vi "FOFB Data Archiver Main.vi"() -> ()   [LabVIEW 2011]
uses:
  Types Definitions/Type BPM and PS select cluster.ctl
  <vilib>/Platform/TimedLoop/XDataNode/timing_clust.ctl
  <vilib>/Platform/TimedLoop/XDataNode/nitl_modes.ctl
  <vilib>/Platform/TimedLoop/XDataNode/wakeup.ctl
  <vilib>/Platform/TimedLoop/XDataNode/XDataNode.xnode
  Type Definitions.lvlib
  Controller VIs.lvlib
  <vilib>/Platform/TimedLoop/XDataNode/XDNodeRunTimeDep.lvlib
  File VIs.lvlib
  kernel32.dll
panel:
  out "Slide":dbl(slide)
  out "Next filename":string caption="Registro de dados em:"
  out "Status":bool caption="Registrando dados..."
  in  "Path":path=path "E:/" caption="Diretório de armazenamento"
  in  "Maximum number of files":i32=18900 caption="Máximo número de arquivos:"
  in  "Number of packets per file":i32=1000 caption="Número de pacotes de dados por arquivo:"
  in  "FOFB Controller IP":string="10.0.5.31" caption="IP do controlador do FOFB (PXI):"
  in  "stop":bool
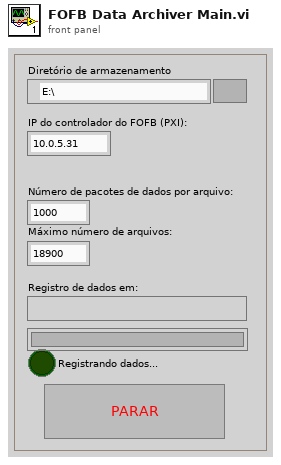
[diagram p1: front panel]
types:
  T1 = typedef "Type Definitions.lvlib/Type BPM and PS select cluster.ctl" = cluster{"BPM index array":u32[], "PS index array ":u32[]}
  T2 = enum16{"Idle", "Wait Connection", "Read Data", "Close Connection"}
  T3 = typedef "XDNodeRunTimeDep.lvlib/timing_clust.ctl" = cluster{"Expected End [f-1]":u64, "Actual End [f-1]":u64, "Finished Late? [f-1]":bool, "Expected End [i-1]":u64, "Actual End [i-1]":u64, "Finished Late? [i-1]":bool, "Expected Start [i]":u64, "Actual Start [i]":u64, "Expected Start [f]":u64, "Actual Start [f]":u64, "Source Name":string, "Structure Name":string, "Period":i64, "Deadline":i64, "Offset":i64, "Start":i64, "Priority":i32, "Timeout":i32, "Mode":T4, "Wakeup Reason":T5, "Error":errorcluster, "Source Type":string, "Secondary Source Type":string, "Global End Time":u64, "Global Start Time":u64, "Frame Duration":u64, "Iteration Duration":u64, "Assigned CPU":i32, "I/O Scan Engine Mode":u32}
  T4 = typedef "XDNodeRunTimeDep.lvlib/nitl_modes.ctl" = enum32{"No Change", "Process missed periods, maintain original phase", "Discard missed periods, maintain original phase", "Process missed periods, ignore original phase", "Discard missed periods, ignore original phase"}
  T5 = typedef "XDNodeRunTimeDep.lvlib/wakeup.ctl" = enum32{"Normal", "Aborted", "Asynchronous wakeup", "Timing source error", "Timed loop error", "Timeout"}
  T6 = enum16{"open", "replace", "create", "open or create", "replace or create", "replace or create with confirmation"}
  T7 = typedef "Type Definitions.lvlib/Type FOFB Parameters.ctl" = cluster{"Network":T8, "Fast Acquisition":T9, "Response Matrix Measurement":T10, "Correction Algorithm":T11, "Acquisition Network":T12, "Actuation Network":T13}
  T8 = typedef "Type Definitions.lvlib/Type Network Configuration.ctl" = cluster{"FOFB Controller IP":string, "LNLS Control Network IP":string, "LNLS Control Network Power Supplies TCP Port":u16, "LNLS Control Network FOFB Configuration TCP Port":u16, "LNLS Control Network BPMs TCP Port":u16, "Data Server TCP Port":u16, "Monitoring Data TCP Port":u16, "Configuration GUI TCP Port":u16, "Storage Data TCP Port":u16, "Fast Command TCP Port":u16, "TCP Listening Timeout":i32, "Request Setpoints Rate":u16}
  T9 = typedef "Type Definitions.lvlib/Type FA Configuration.ctl" = cluster{"Acquisition Period":u32, "Data Buffer Size":u32, "Monitoring Period":u32}
  T10 = typedef "Type Definitions.lvlib/Type Response Matrix Measurement Configuration.ctl" = cluster{"Step Amplitude":dbl, "Time Between Steps":u32, "Step Duration":u32, "Number of Averages":u32}
  T11 = typedef "Type Definitions.lvlib/Type Correction Algorithm Configuration.ctl" = cluster{"Correction Period":u32, "Reference Orbit Path":path, "Response Matrix Path":path, "Correction Matrix Path":path, "PID Horizontal Gain":dbl, "PID Vertical Gain":dbl, "PID Horizontal Integral Time":dbl, "PID Vertical Integral Time":dbl, "PID Horizontal Derivative Time":dbl, "PID Vertical Derivative Time":dbl, "Beam Current FOFB Threshold":dbl, "Decouple H-V":bool, "Use Additional BPM LPF":bool, "BPM LPF Cutoff":dbl}
  T12 = typedef "Type Definitions.lvlib/Type Acquisition Network Configuration.ctl" = cluster{"Chassis Name":string, "Variables":cluster{"Variable Name":string, "Matrix Order":u32, "Location":dbl, "Plane":enum8{"H", "V"}, "On Correction":bool}[]}[]
  T13 = typedef "Type Definitions.lvlib/Type Actuation Network Configuration.ctl" = cluster{"Chassis Name":string, "Variables":cluster{"Variable Name":string, "Matrix Order":u32, "RMM Step Factor":dbl, "Plane":enum8{"H", "V"}, "On Correction":bool, "Kc":dbl, "Ti":dbl, "Td":dbl}[]}[]
  T14 = typedef "Type Definitions.lvlib/Type FOFB Configuration.ctl" = cluster{"FOFB Parameters":T7, "Number of Acquisition Chassis":i32, "Number of Actuation Chassis":i32, "Number of BPM Readings":i32, "BPM Reading Names":string[], "Selected BPM Readings":u32[], "Number of Correctors":i32, "Corrector Names":string[], "Selected Correctors":u32[], "Reference Orbit":dbl[], "Response Matrix":dbl[][], "Correction Matrix":dbl[][], "Acquisition Chassis Names":string[], "Actuation Chassis Names":string[], "Acquisition Variables":cluster{"Variable Name":string, "Chassis Name":string}[], "Actuation Variables":cluster{"Variable Name":string, "Chassis Name":string}[], "PS Matrix Mapping":cluster{u32[]}[], "Inverse PS Matrix Mapping":u32[][], "BPM Matrix Mapping":cluster{u32[]}[], "Inverse BPM Matrix Mapping":u32[][], "Response Matrix Beam Energy (MeV)":dbl, "PID Parameters":T15[], "BPM Planes":enum8{"H", "V"}[], "Corrector Planes":enum8{"H", "V"}[], "RMM Step Factor":dbl[]}
  T15 = typedef "Type Definitions.lvlib/Type PID Parameters.ctl" = cluster{"Kc":fxp<+/-,16,8>, "Ti":fxp<+/-,16,8>, "Td":fxp<+/-,16,8>}
  T16 = enum16{"Standard", "Buffered", "CRLF", "Immediate"}
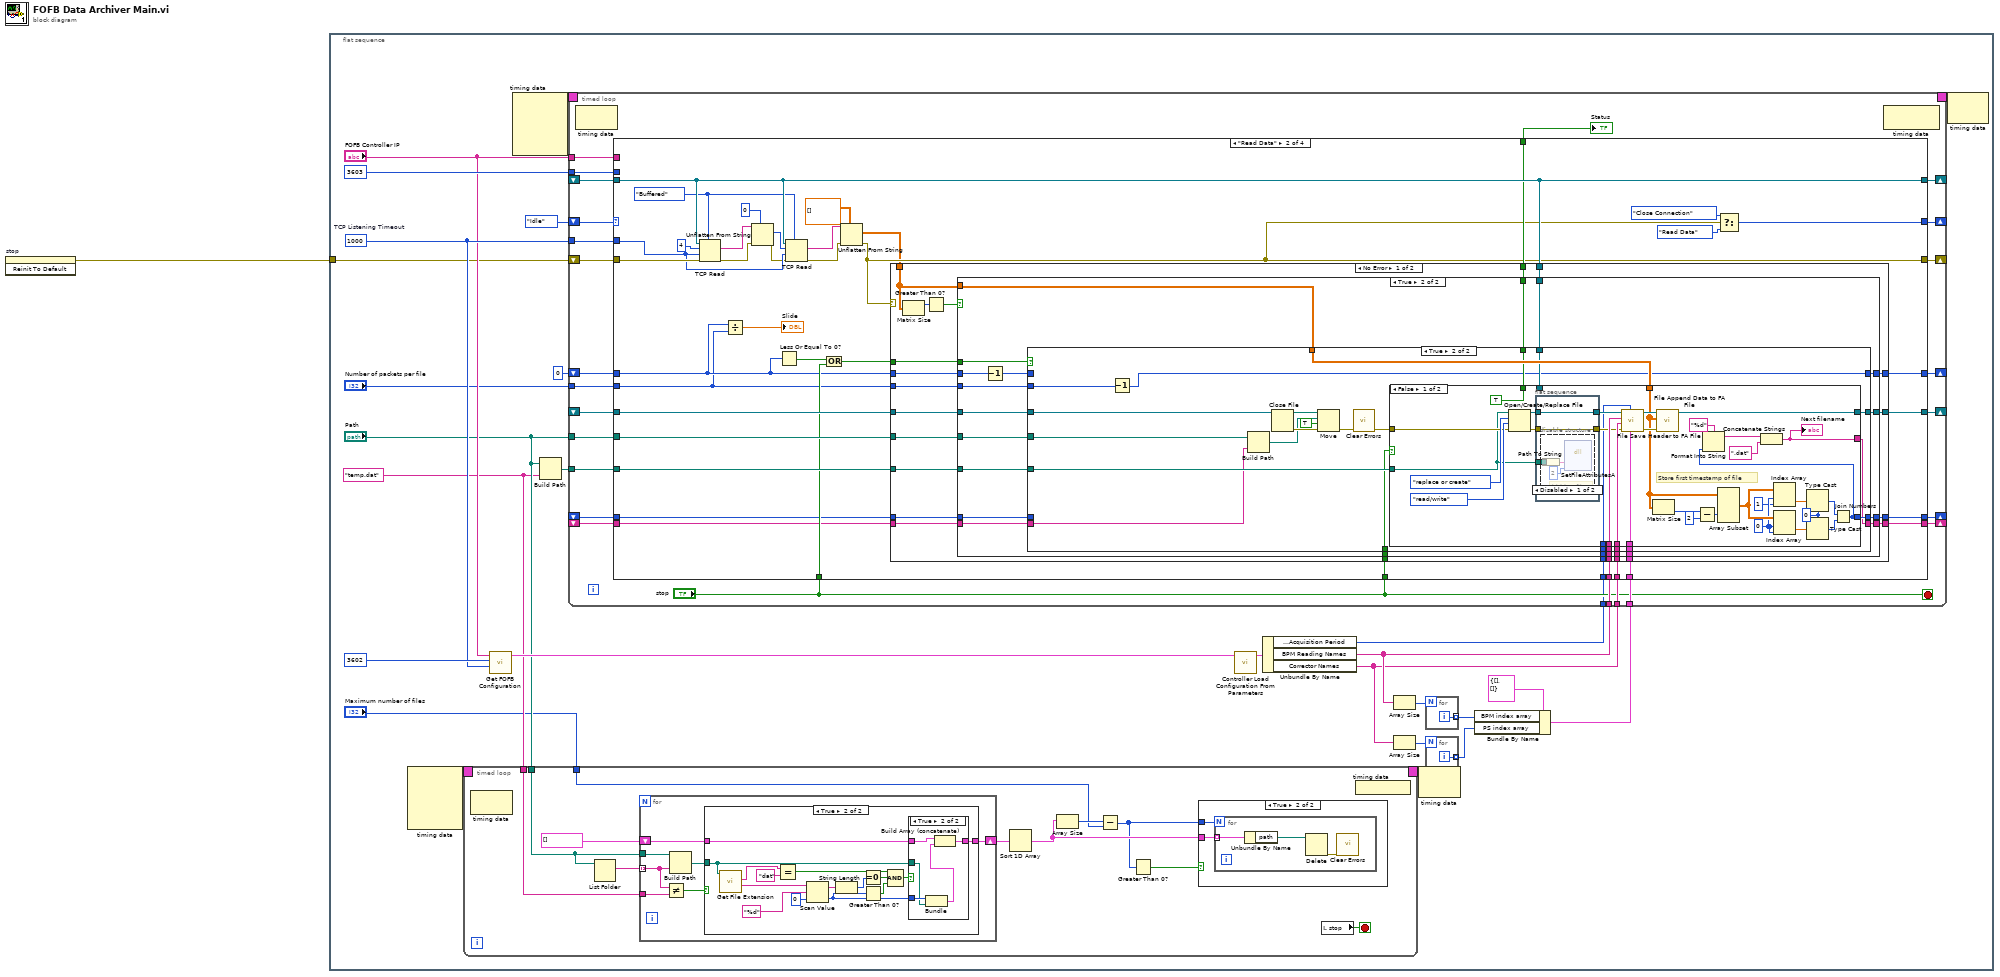
[diagram p0: block diagram]
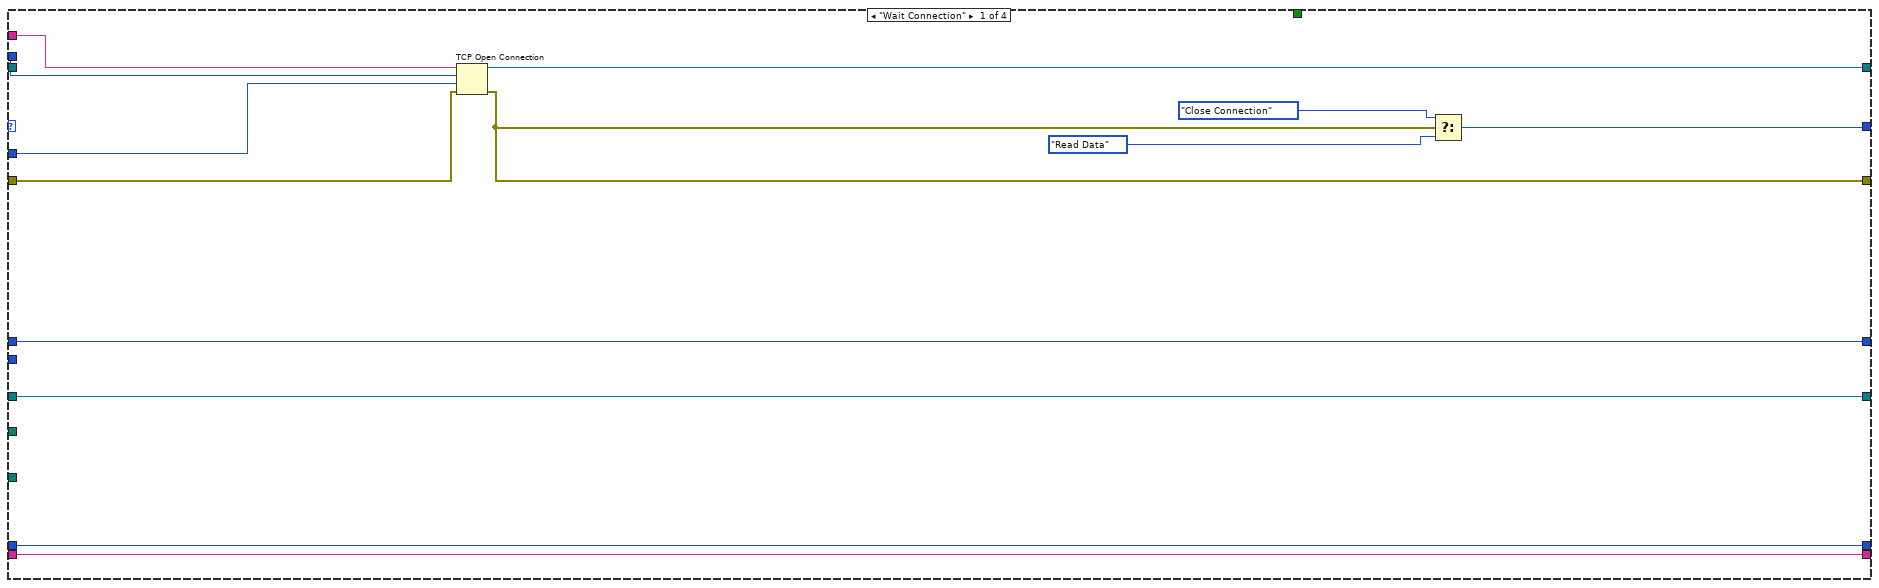
[diagram p2: hidden frame]
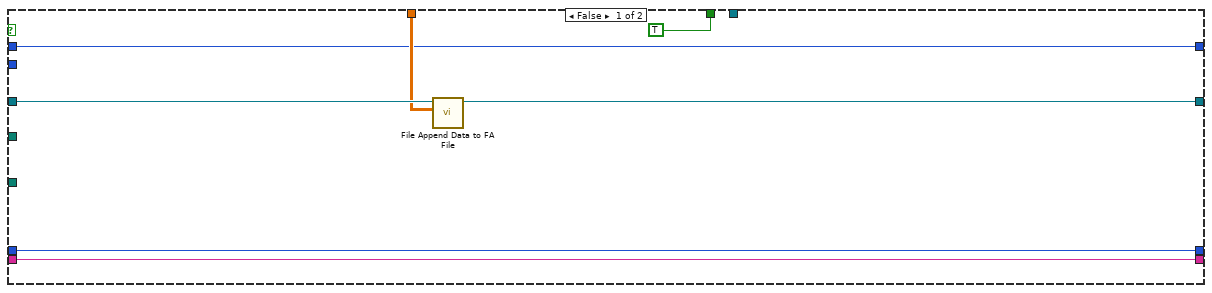
[diagram p4: hidden frame]
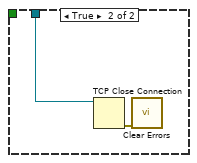
[diagram p6: hidden frame]
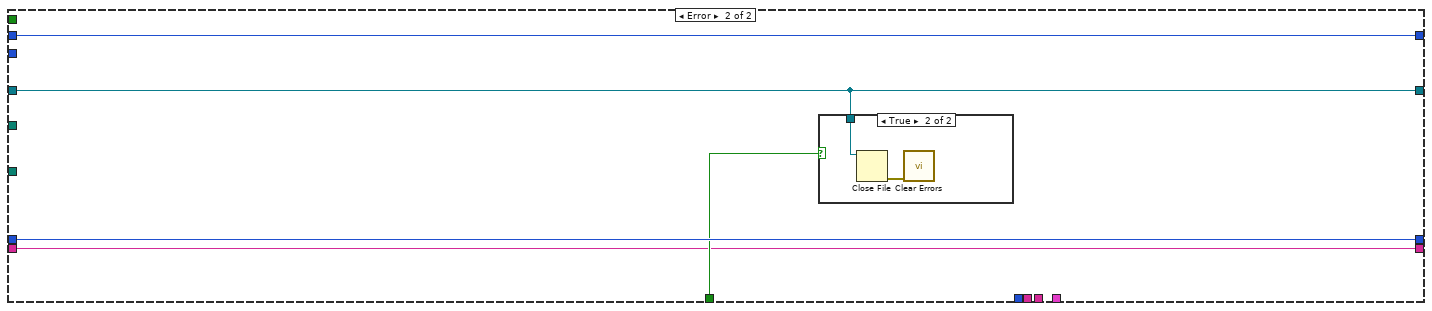
[diagram p7: hidden frame]
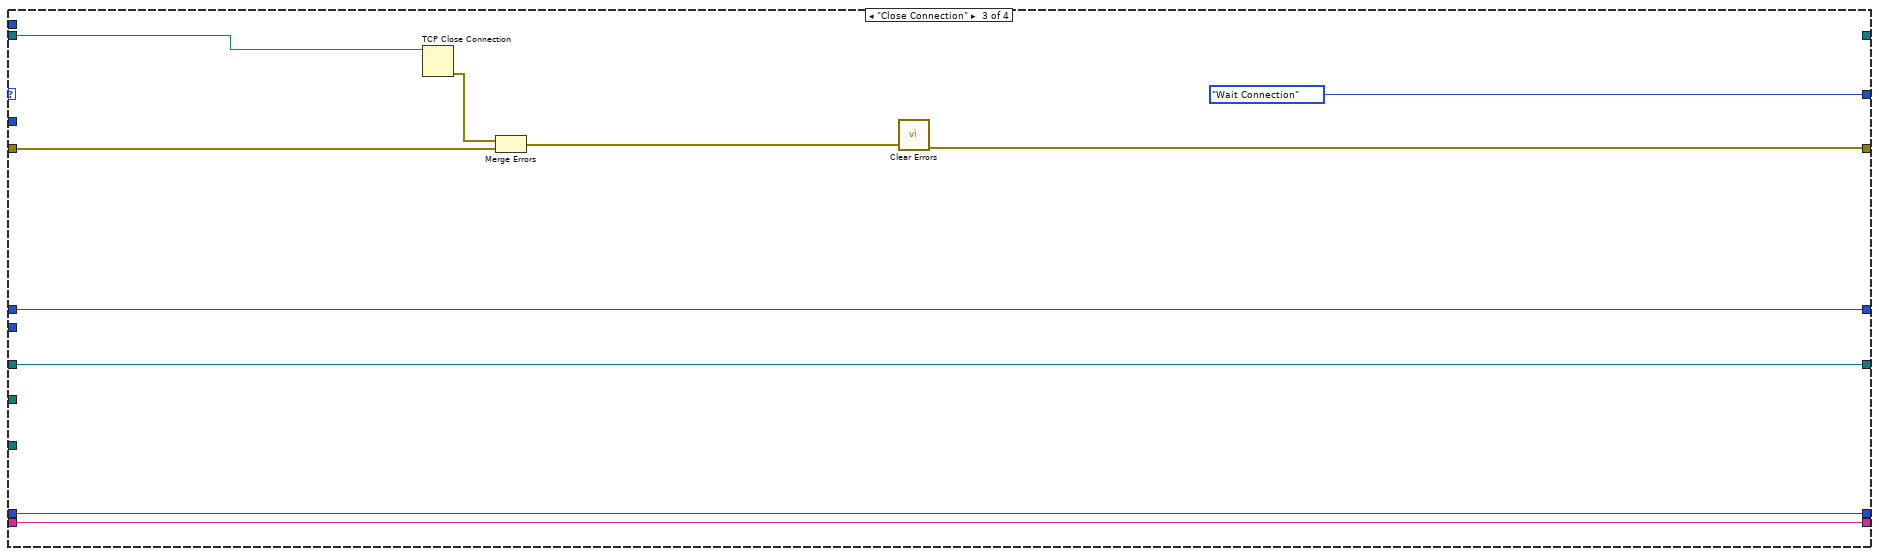
[diagram p9: hidden frame]
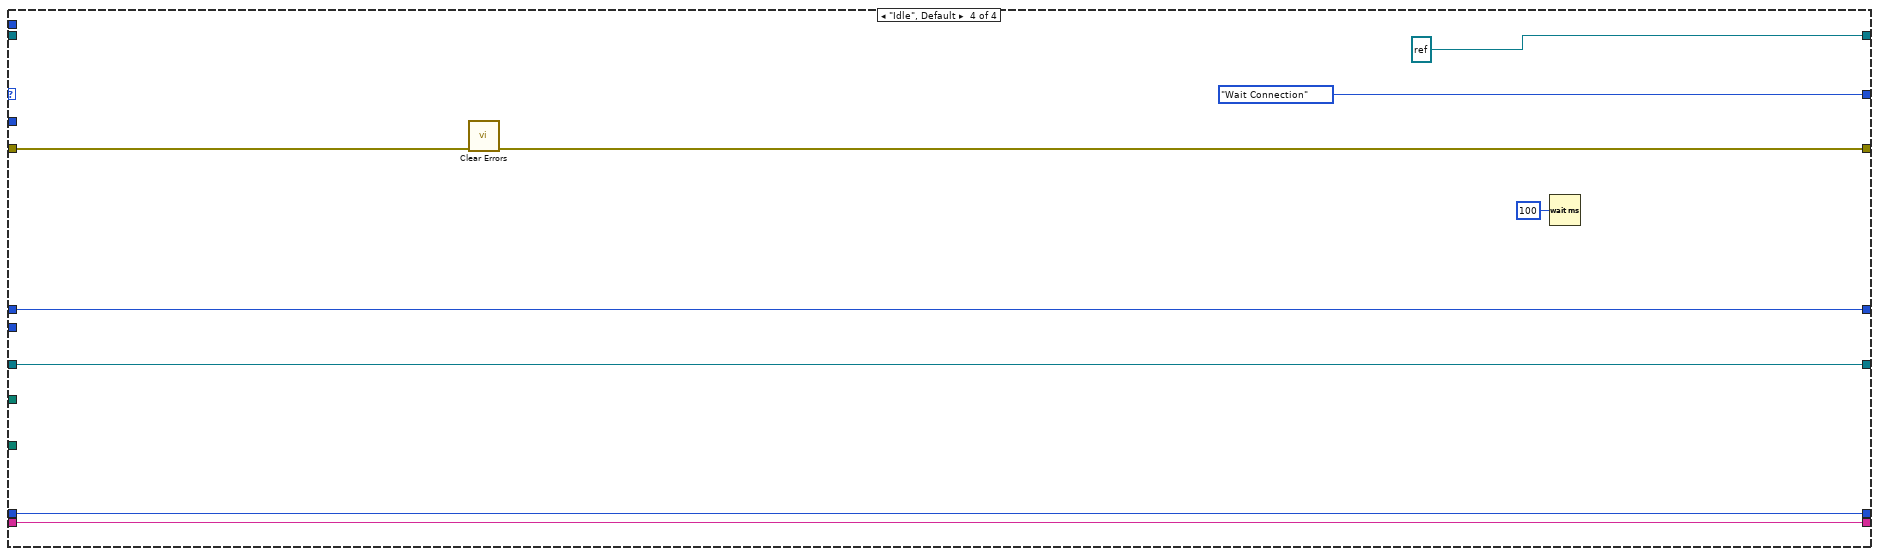
[diagram p10: hidden frame]
diagram:
  n1 = invoke on="stop" class="Bool (strict)" method="Reinit To Default"() -> (error out=w1:errorcluster)  [unwired: 3 in, 2 out]
  n2 = flat-sequence {
    tunnel: w1 -> [w7]
    frame #0 {
      w9 = "temp.dat" ("FOFB Controller IP")
      w16 = 1000  # TCP Listening Timeout
      n3 = node-c288() -> (w28:T3)  [unwired: 4 in]
      n4 = timed-loop {
        timing: w28 -> [_]
        timing-out: [_] -> w27
        tunnel: "Path" -> [w258]
        tunnel: w9 -> [w260]
        tunnel: "Maximum number of files" -> [w259]
        stop <- w261 stop-if-true
        n5 = node-c288() -> ()  [unwired: 1 in, 1 out]
        n6 = List Folder(path=w258) -> (filenames=w265:string[])  [unwired: 3 in, 3 out]
        n7 = for {
          tunnel: w258 -> [w277]
          tunnel: w265 -> [w272] mode=indexing
          shift-right: [w276] -> w263
          shift-left: cluster{"timestamp":u64, "path":path}[] [] -> [w274]
          tunnel: w260 -> [w271]
          n8 = Not Equal?(x=w272, y=w271) -> (x != y?=w273:bool)
          n9 = Build Path(base path=w277, name or relative path=w272) -> (appended path=w275:path)
          n10 = case shown="True" w273 {
            tunnel: [w278 w293] -> w276
            tunnel: w275 -> [_ w290]
            tunnel: w274 -> [w278 w292]
            frame False {
            }
            frame True {
              n11 = call <vilib>:"Get File Extension.vi"("file"=w290) -> ("filename without extension"=w288:string, "lowercase file extension"=w289:string)  [unwired: 7 in, 2 out]
              n12 = Equal?(x=w289, y="dat") -> (x = y?=w286:bool)
              n13 = Scan Value(string=w288, format string="%d", default (0 dbl)=u64 0 ("const")) -> (output string=w279:string, value=w283:u64)
              n14 = String Length(string=w279) -> (length=w280:i32)
              n15 = Equal To 0?(x=w280) -> (x = 0?=w281:bool)
              n16 = Greater Than 0?(x=w283) -> (x > 0?=w282:bool)
              n17 = Compound Arithmetic op=AND(w286, w281, w282) -> (w285:bool)
              n18 = case shown="True" w285 {
                tunnel: w292 -> [w294 w299]
                tunnel: [w294 w298] -> w293
                tunnel: w290 -> [_ w295]
                tunnel: w283 -> [_ w296]
                frame False {
                }
                frame True {
                  n19 = Bundle("const"=w296, "appended path"=w295) -> (w297:cluster{"const":u64, "appended path":path})  [unwired: 1 in]
                  n20 = Build Array (concatenate)(w299, w297) -> (w298:cluster{"const":u64, "appended path":path}[])
                }
              }
            }
          }
        }
        n21 = Sort 1D Array(array=w263) -> (sorted array=w257:cluster{"timestamp":u64, "path":path}[])
        n22 = Array Size(array=w257) -> (size(s)=w262:i32)
        n23 = Subtract(x=w262, y=w259) -> (x-y=w256:i32)
        n24 = Greater Than 0?(x=w256) -> (x > 0?=w255:bool)
        n25 = case shown="True" w255 {
          tunnel: w257 -> [_ w266]
          tunnel: w256 -> [_ w267]
          frame False {
          }
          frame True {
            n26 = for {
              N: w267 -> [_]
              tunnel: w266 -> [w270] mode=indexing
              n27 = Unbundle By Name(w270) -> ("path"=w269:path)
              n28 = Delete(path (use dialog)=w269) -> (error out=w268:errorcluster)  [unwired: 4 in, 2 out]
              n29 = call <vilib>:"Clear Errors.vi"("error in (no error)"=w268) -> ()  [unwired: 6 in, 1 out]
            }
          }
        }
        n30 = local read "stop"() -> (w261:bool)
        n31 = node-c288() -> ()  [unwired: 1 out]
      }
      n32 = call "Get FOFB Configuration.vi"("TCP Listening Timeout"=w16, "Configuration TCP Port"=u16 3602 ("Configuration GUI TCP Port"), "FOFB Controller IP"="FOFB Controller IP") -> ("FOFB Parameters"=w14:T7)  [unwired: 7 in, 1 out]
      n33 = node-c288() -> (w3:T3)  [unwired: 4 in]
      n34 = Build Path(base path="Path", name or relative path=w9) -> (appended path=w24:path)
      n35 = call "Controller Load Configuration From Parameters.vi"("FOFB Parameters"=w14) -> ("FOFB Configuration"=w13:T14)  [unwired: 9 in, 1 out]
      n36 = Unbundle By Name(w13) -> ("FOFB Parameters.Fast Acquisition.Acquisition Period"=w6:u32, "BPM Reading Names"=w12:string[], "Corrector Names"=w11:string[])
      n37 = Array Size(array=w12) -> (size(s)=w23:i32)
      n38 = Array Size(array=w11) -> (size(s)=w19:i32)
      n39 = node-c288(w27) -> ()  [unwired: 1 out]
      n40 = for {
        N: w23 -> [_]
        tunnel: [w305] -> w20 mode=indexing
        i -> [w305]
      }
      n41 = for {
        N: w19 -> [_]
        tunnel: [w304] -> w18 mode=indexing
        i -> [w304]
      }
      n42 = Bundle By Name(cluster=T1 {"BPM index array"=[], "PS index array "=[]} ("BPM and PS selection"), "BPM index array"=w20, "PS index array"=w18) -> (w22:T1)
      n43 = timed-loop {
        shift-right: [w46] -> _
        shift-left: w7 -> [w54]
        shift-right: [w50] -> _
        shift-left: T2."Idle" ("f") -> [w52]
        shift-right: [w51] -> _
        shift-left: _ -> [w53]
        tunnel: "FOFB Controller IP" -> [w49]
        tunnel: u16 3603 ("TCP Port") -> [w48]
        tunnel: w16 -> [w47]
        shift-right: [w44] -> _
        shift-left: 0 ("Number of packets per file") -> [w45]
        tunnel: "Number of packets per file" -> [w43]
        shift-right: [w42] -> _
        shift-left: _ -> [w41]
        tunnel: w24 -> [w40]
        tunnel: "Path" -> [w39]
        tunnel: w12 -> [w38]
        tunnel: w11 -> [w37]
        tunnel: w22 -> [w36]
        tunnel: w6 -> [w33]
        shift-right: [w31] -> _
        shift-left: _ -> [w32]
        shift-right: [w30] -> _
        shift-left: _ -> [w29]
        timing: w3 -> [_]
        timing-out: [_] -> w2
        stop <- "stop" stop-if-true
        n44 = node-c288() -> ()  [unwired: 1 in, 1 out]
        n45 = case shown="\"Read Data\"" w52 {
          tunnel: [w69 w85 _ refnum<k5> refnum ("connection ID")] -> w51
          tunnel: [w68 w108 T2."Wait Connection" ("f") T2."Wait Connection" ("f")] -> w50
          tunnel: [w62 w78 w238 w249] -> w46
          tunnel: w54 -> [w67 w107 w240 w250]
          tunnel: w53 -> [_ w85 w243 _]
          tunnel: w49 -> [w64 _ _ _]
          tunnel: w48 -> [w63 _ _ _]
          tunnel: w47 -> [w61 w98 _ _]
          tunnel: w45 -> [w58 w72 w235 w245]
          tunnel: [w58 w97 w235 w245] -> w44
          tunnel: w43 -> [_ w71 _ _]
          tunnel: [w60 w96 w237 w247] -> w42
          tunnel: w41 -> [w60 w95 w237 w247]
          tunnel: w40 -> [_ w94 _ _]
          tunnel: w39 -> [_ w93 _ _]
          tunnel: "stop" -> [_ w92 _ _]
          tunnel: "stop" -> [_ w89 _ _]
          tunnel: w38 -> [_ w88 _ _]
          tunnel: w37 -> [_ w87 _ _]
          tunnel: w36 -> [_ w86 _ _]
          tunnel: [_ w84 _ _] -> w34
          tunnel: w33 -> [_ w83 _ _]
          tunnel: w32 -> [w59 w77 w236 w246]
          tunnel: [w59 w82 w236 w246] -> w31
          tunnel: [w57 w75 w234 w244] -> w30
          tunnel: w29 -> [w57 w74 w234 w244]
          frame "Wait Connection" {
            n46 = TCP Open Connection(address=w64, remote port or service name=w63, timeout ms (60000)=w61, error in (no error)=w67) -> (connection ID=w69:refnum<k5>, error out=w62:errorcluster)  [unwired: 1 in]
            n47 = Select(t=T2."Close Connection" ("f"), s=w62, f=T2."Read Data") -> (s? t:f=w68:T2)
          }
          frame "Read Data" {
            w76 = T16."Buffered" ("mode (standard)")
            n48 = TCP Read(connection ID=w85, bytes to read=4, error in (no error)=w107, 7:w76, 9:w98) -> (data out=w103:string, error out=w81:errorcluster)  [unwired: 1 out]
            n49 = Divide(x=w72, y=w71) -> (x/y=→"Slide":dbl)
            n50 = Unflatten From String(type=0 ("bytes to read"), binary string=w103, error in (no error)=w81) -> (value=w101:i32, error out=w80:errorcluster)  [unwired: 2 in, 1 out]
            n51 = Less Or Equal To 0?(x=w72) -> (x <= 0?=w90:bool)
            n52 = TCP Read(connection ID=w85, bytes to read=w101, error in (no error)=w80, 7:w76, 9:w98) -> (data out=w100:string, error out=w79:errorcluster)  [unwired: 1 out]
            n53 = Or(x=w90, y=w92) -> (x .or. y?=w91:bool)
            n54 = Unflatten From String(type=sgl[][] [] ("BPM and PS Data"), binary string=w100, error in (no error)=w79) -> (value=w70:sgl[][], error out=w78:errorcluster)  [unwired: 2 in, 1 out]
            n55 = case shown="No Error" w78 {
              tunnel: [w130 w231] -> w97
              tunnel: w71 -> [w129 _]
              tunnel: w72 -> [w112 w231]
              tunnel: w70 -> [w114 _]
              tunnel: [w128 w228] -> w96
              tunnel: w95 -> [w127 w228]
              tunnel: w94 -> [w126 _]
              tunnel: w93 -> [w125 _]
              tunnel: w91 -> [w124 _]
              tunnel: w89 -> [w123 w229]
              tunnel: w88 -> [w122 _]
              tunnel: w87 -> [w121 _]
              tunnel: w86 -> [w120 _]
              tunnel: w85 -> [w119 _]
              tunnel: [w118 _] -> w84
              tunnel: w83 -> [w117 _]
              tunnel: w77 -> [w116 w230]
              tunnel: [w115 w230] -> w82
              tunnel: [w110 w227] -> w75
              tunnel: w74 -> [w109 w227]
              frame No Error {
                n56 = Matrix Size(0:w114) -> (1:w113:i32)  [unwired: 1 out]
                n57 = Greater Than 0?(x=w113) -> (x > 0?=w111:bool)
                n58 = case shown="True" w111 {
                  tunnel: [w132 w140] -> w130
                  tunnel: w129 -> [_ w155]
                  tunnel: w112 -> [w132 w139]
                  tunnel: [w134 w154] -> w128
                  tunnel: w127 -> [w134 w153]
                  tunnel: w126 -> [_ w152]
                  tunnel: w125 -> [_ w151]
                  tunnel: w124 -> [_ w138]
                  tunnel: w123 -> [_ w150]
                  tunnel: w122 -> [_ w149]
                  tunnel: w121 -> [_ w148]
                  tunnel: w120 -> [_ w147]
                  tunnel: w119 -> [_ w146]
                  tunnel: [_ w145] -> w118
                  tunnel: w117 -> [_ w144]
                  tunnel: w116 -> [w133 w143]
                  tunnel: [w133 w142] -> w115
                  tunnel: w114 -> [_ w141]
                  tunnel: [w131 w137] -> w110
                  tunnel: w109 -> [w131 w136]
                  frame False {
                  }
                  frame True {
                    n59 = Decrement(x=w139) -> (x-1=w135:i32)
                    n60 = case shown="True" w138 {
                      tunnel: [w157 w165] -> w140
                      tunnel: w155 -> [_ w166]
                      tunnel: w141 -> [w158 w176]
                      tunnel: [w162 w178] -> w154
                      tunnel: w153 -> [w161 w185]
                      tunnel: w152 -> [_ w184]
                      tunnel: w151 -> [_ w183]
                      tunnel: w143 -> [w160 _]
                      tunnel: [w160 w175] -> w142
                      tunnel: w150 -> [_ w174]
                      tunnel: w149 -> [_ w173]
                      tunnel: w148 -> [_ w172]
                      tunnel: w147 -> [_ w171]
                      tunnel: w146 -> [_ w170]
                      tunnel: [TRUE ("stop 2") w169] -> w145
                      tunnel: w144 -> [_ w168]
                      tunnel: w135 -> [w157 _]
                      tunnel: [w156 w164] -> w137
                      tunnel: w136 -> [w156 w163]
                      frame False {
                        n61 = call "File Append Data to FA File.vi"("Data"=w158, "FA File Reference"=w161) -> ("FA File Reference"=w162:refnum<file>)  [unwired: 7 in, 1 out]
                      }
                      frame True {
                        n62 = Decrement(x=w166) -> (x-1=w165:i32)
                        n63 = Build Path(base path=w183, name or relative path=w163) -> (appended path=w180:path)
                        n64 = Close File(refnum=w185) -> (path=w181:path, error out=w182:errorcluster)  [unwired: 1 in]
                        n65 = Move(source path=w181, error in=w182, 9:TRUE ("overwrite (F)"), 10:w180) -> (error out=w167:errorcluster)  [unwired: 1 in, 2 out]
                        n66 = call <vilib>:"Clear Errors.vi"("error in (no error)"=w167) -> ("error out"=w177:errorcluster)  [unwired: 6 in]
                        n67 = case shown="False" w174 {
                          tunnel: w184 -> [w207 _]
                          tunnel: [w216 _] -> w178
                          tunnel: w177 -> [w213 _]
                          tunnel: w176 -> [w212 _]
                          tunnel: [w187 _] -> w175
                          tunnel: w173 -> [w210 _]
                          tunnel: w172 -> [w209 _]
                          tunnel: w171 -> [w208 _]
                          tunnel: w170 -> [_ w226]
                          tunnel: [TRUE ("stop 2") _] -> w169
                          tunnel: w168 -> [w201 _]
                          tunnel: [w186 _] -> w164
                          frame False {
                            w198 = u32 0
                            w192 = 0 ("row 1")
                            # "Store first timestamp of file"
                            n68 = Open/Create/Replace File(file path (use dialog)=w207, error in=w213, operation (0:open)=T6."replace or create", access (0:read/write)=enum16{"read/write", "read-only", "write-only"}."read/write") -> (refnum out=w203:refnum<file>, error out=w205:errorcluster)  [unwired: 2 in, 1 out]
                            n69 = flat-sequence {
                              tunnel: w207 -> [w221]
                              tunnel: [w220] -> w206
                              tunnel: w205 -> [w220]
                              tunnel: [w219] -> w204
                              tunnel: w203 -> [w219]
                              frame #0 {
                                n70 = disable-structure shown="Disabled" {
                                disable-tunnel: w221 -> [w223 _]
                                frame Disabled {
                                # "hidden file"
                                n71 = Path To String(path=w223) -> (string=w222:string)
                                n72 = dll-call lib="kernel32.dll" fn="SetFileAttributesA"("lpFileName"=w222, "dwFileAttributes"=u32 2) -> ()  [unwired: 6 in, 2 out]
                                }
                                frame Enabled {
                                }
                                }
                              }
                            }
                            n73 = call "File Save Header to FA File.vi"("BPM and PS selection"=w208, "Acquisition period (us)"=w201, "error in (no error)"=w206, "PS Reading Names"=w209, "BPM Reading Names"=w210, "FA File Reference"=w204) -> ("error out"=w215:errorcluster, "FA File Reference out"=w214:refnum<file>)  [unwired: 4 in]
                            n74 = Matrix Size(0:w212) -> (2:w200:i32)  [unwired: 1 out]
                            n75 = call "File Append Data to FA File.vi"("error in (no error)"=w215, "Data"=w212, "FA File Reference"=w214) -> ("FA File Reference"=w216:refnum<file>)  [unwired: 6 in, 1 out]
                            n76 = Subtract(x=w200, y=2) -> (x-y=w211:i32)
                            n77 = Array Subset(array=w212, index (col)=w211) -> (w196:sgl[][])  [unwired: 3 in]
                            n78 = Index Array(array=w196, index (row)=w192, index (col)=1) -> (element=w195:sgl)
                            n79 = Index Array(array=w196, index (row)=w192, index (col)=w192) -> (element=w197:sgl)
                            n80 = Type Cast(type=w198, x=w195) -> (*(type *) &x=w194:u32)
                            n81 = Type Cast(type=w198, x=w197) -> (*(type *) &x=w193:u32)
                            n82 = Join Numbers(hi=w194, lo=w193) -> ((hi.lo)=w187:u64)
                            n83 = Format Into String(format string="%d", w187) -> (resulting string=w190:string)  [unwired: 2 in, 1 out]
                            n84 = Concatenate Strings(w190, ".dat" ("time format string (%c)")) -> (w186:string)
                            "Next filename" <- w186
                          }
                          frame True {
                            n85 = TCP Close Connection(connection ID=w226) -> (error out=w225:errorcluster)  [unwired: 2 in, 1 out]
                            n86 = call <vilib>:"Clear Errors.vi"("error in (no error)"=w225) -> ()  [unwired: 6 in, 1 out]
                          }
                        }
                      }
                    }
                  }
                }
              }
              frame Error {
                n87 = case shown="True" w229 {
                  tunnel: w228 -> [_ w233]
                  frame False {
                  }
                  frame True {
                    n88 = Close File(refnum=w233) -> (error out=w232:errorcluster)  [unwired: 1 in, 1 out]
                    n89 = call <vilib>:"Clear Errors.vi"("error in (no error)"=w232) -> ()  [unwired: 6 in, 1 out]
                  }
                }
              }
            }
            n90 = Select(t=T2."Close Connection" ("f"), s=w78, f=T2."Read Data") -> (s? t:f=w108:T2)
          }
          frame "Close Connection" {
            n91 = TCP Close Connection(connection ID=w243) -> (error out=w241:errorcluster)  [unwired: 2 in, 1 out]
            n92 = Merge Errors(w241, w240) -> (w239:errorcluster)
            n93 = call <vilib>:"Clear Errors.vi"("error in (no error)"=w239) -> ("error out"=w238:errorcluster)  [unwired: 6 in]
          }
          frame "Idle", Default {
            n94 = call <vilib>:"Clear Errors.vi"("error in (no error)"=w250) -> ("error out"=w249:errorcluster)  [unwired: 6 in]
            n95 = Wait (ms)(milliseconds to wait=u32 100 ("millisecond multiple")) -> ()  [unwired: 1 out]
          }
        }
        "Status" <- w34
        n96 = node-c288() -> ()  [unwired: 1 in, 1 out]
      }
      n97 = node-c288(w2) -> ()  [unwired: 1 out]
    }
  }
